vi "Attempt-create-client.vi"(8 "error in (no error)":errorcluster, 9 "Module path":path, 10 "Module type":string, 11 "ModComm in":T1) -> (0 "error out":errorcluster, 3 "ModComm out":T1)   [LabVIEW 2013, in "Server.lvlib" / "Server.lvclass"]
uses:
  Server.lvclass
  Object-reference.ctl
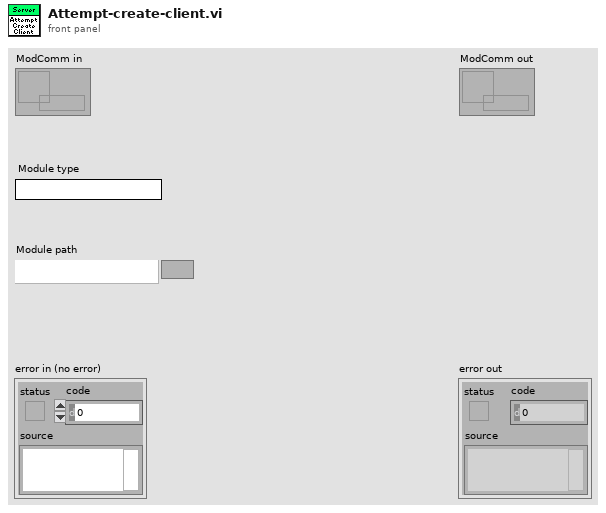
[diagram p1: front panel]
types:
  T1 = typedef "Server.lvlib/Server.lvclass/Object-reference.ctl" = refnum<data-value>
  T2 = typedef "Server.lvlib/Server.lvclass/Supported-module-types.ctl" = enum16{"Server", "All", "BeamControl", "PowderDeposition", "StrategyParser", "CameraVision", "MaterialCharacterization", "StatusMonitor", "SLMSimulation", "LaserCharacterization"}
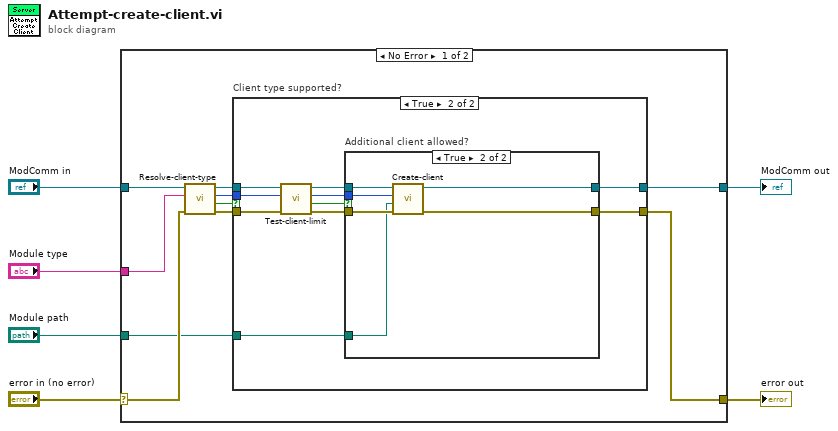
[diagram p0: block diagram]
diagram:
  n1 = case shown="No Error" "error in (no error)" {
    selector: "error in (no error)" -> [w10 w38]
    tunnel: [w8 w38] -> w5
    tunnel: [w9 w37] -> w3
    tunnel: "ModComm in" -> [w16 w37]
    tunnel: "Module type" -> [w15 _]
    tunnel: "Module path" -> [w7 _]
    frame No Error {
      n2 = call "Resolve-client-type.vi"("error in (no error)"=w10, "Module name"=w15, "ModComm in"=w16) -> ("error out"=w11:errorcluster, "Supported?"=w13:bool, "Module type"=w12:T2, "ModComm out"=w14:T1)  [unwired: 5 in]
      n3 = case "Client type supported?" shown="True" w13 {
        tunnel: w14 -> [w18 w28]
        tunnel: w12 -> [_ w26]
        tunnel: w11 -> [w17 w27]
        tunnel: [w18 w21] -> w9
        tunnel: [w17 w20] -> w8
        tunnel: w7 -> [_ w19]
        frame False {
        }
        frame True {
          n4 = call "Test-client-limit.vi"("error in (no error)"=w27, "Module type"=w26, "ModComm in"=w28) -> ("error out"=w24:errorcluster, "Client allowed?"=w25:bool, "Module type dup"=w22:T2, "ModComm out"=w23:T1)  [unwired: 5 in]
          n5 = case "Additional client allowed?" shown="True" w25 {
            tunnel: w24 -> [w29 w34]
            tunnel: w23 -> [w30 w36]
            tunnel: w22 -> [_ w32]
            tunnel: [w30 w35] -> w21
            tunnel: [w29 w33] -> w20
            tunnel: w19 -> [_ w31]
            frame False {
            }
            frame True {
              n6 = call "Create-client.vi"("error in (no error)"=w34, "Module path"=w31, "Module type"=w32, "ModComm in"=w36) -> ("error out"=w33:errorcluster, "ModComm out"=w35:T1)  [unwired: 6 in]
            }
          }
        }
      }
    }
    frame Error {
    }
  }
  "error out" <- w5
  "ModComm out" <- w3
